vi "hwOperation_GetMeasurementValue.vi"(7 "hwType":string, 8 "Error in":errorcluster, 11 "hwDriverRef in":T1) -> (0 "Error out":errorcluster, 1 "Waveform[]":waveform(dbl)[](array[waveform]), 2 "Time Stamp":timestamp, 3 "hwDriverRef out":T1, 4 "Cluster":cluster{i32[], i32[]}, 5 "Values":dbl[](array[numeric]))   [LabVIEW 2016]
uses:
  QX/hw_QX_hwDriverRef.ctl
  C:/Users/CL/Desktop/ZcDAQprj0811/ZcDAQprj/Modules/DAQ-Device/Hardware Drivers/QX/HBM LabVIEW Driver/DLLs/Hbm.Api.Common.dll
  QX/HBM LabVIEW Driver/DLLs/Hbm.Api.Common.dll
panel:
  in  "Index":i32
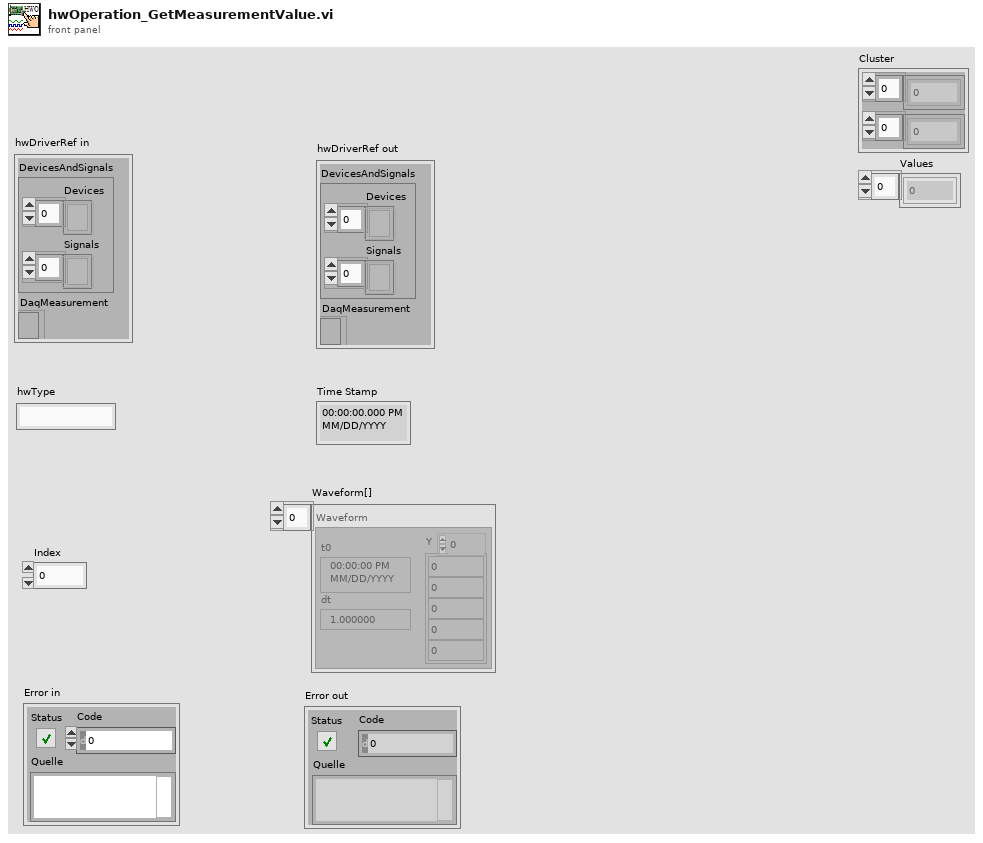
[diagram p1: front panel]
types:
  T1 = typedef "hw_QX_hwDriverRef.ctl" = cluster{"DevicesAndSignals":cluster{"Devices":refnum<k24>[], "Signals":refnum<k24>[]}, "DaqMeasurement":refnum<k24>}
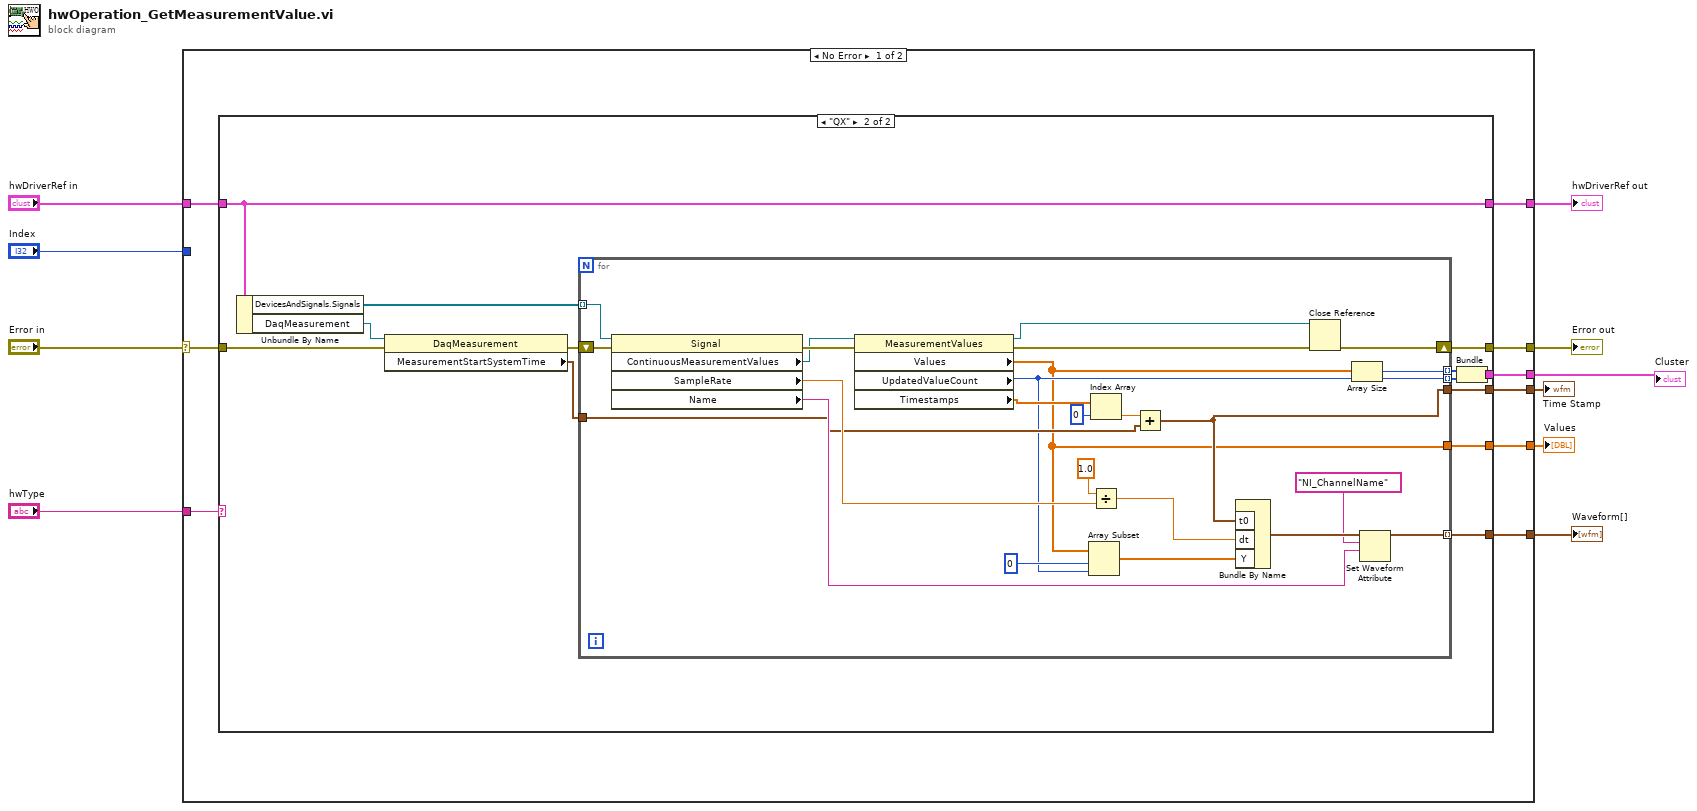
[diagram p0: block diagram]
diagram:
  n1 = case shown="No Error" "Error in" {
    selector: "Error in" -> [w18 w60]
    tunnel: "hwDriverRef in" -> [w19 w59]
    tunnel: [w16 w60] -> w9
    tunnel: [w14 w59] -> w8
    tunnel: "Index" -> [_ _]
    tunnel: [w17 _] -> w6
    tunnel: "hwType" -> [w15 _]
    tunnel: [w13 _] -> w3
    tunnel: [w12 _] -> w2
    tunnel: [w11 _] -> w1
    frame No Error {
      n2 = case shown="\"QX\"" w15 {
        tunnel: w19 -> [w20 w28]
        tunnel: w18 -> [w21 w34]
        tunnel: [_ w32] -> w17
        tunnel: [w21 w31] -> w16
        tunnel: [w20 w28] -> w14
        tunnel: [_ w27] -> w13
        tunnel: [_ w24] -> w12
        tunnel: [_ w23] -> w11
        frame "Simulation", Default {
        }
        frame "QX" {
          n3 = Unbundle By Name(w28) -> ("DevicesAndSignals.Signals"=w30:refnum<k24>[], "DaqMeasurement"=w29:refnum<k24>)
          n4 = property on="Eigenschaftsknoten" class="DaqMeasurement"(reference=w29, error in=w34) -> (error out=w33:errorcluster, "MeasurementStartSystemTime"=w22:timestamp)  [unwired: 1 out]
          n5 = for {
            tunnel: [w48] -> w32 mode=indexing
            shift-right: [w44] -> w31
            shift-left: w33 -> [w50]
            tunnel: w30 -> [w42] mode=indexing
            tunnel: w22 -> [w40]
            tunnel: [w38] -> w27
            tunnel: [w36] -> w26 mode=indexing
            tunnel: [w37] -> w25 mode=indexing
            tunnel: [w35] -> w23
            n6 = property on="Eigenschaftsknoten" class="Signal"(reference=w42, error in=w50) -> (error out=w58:errorcluster, "ContinuousMeasurementValues"=w45:refnum<k24>, "SampleRate"=w55:dbl, "Name"=w47:string)  [unwired: 1 out]
            n7 = property on="Eigenschaftsknoten" class="MeasurementValues"(reference=w45, error in=w58) -> (reference out=w43:refnum<k24>, error out=w46:errorcluster, "Values"=w35:dbl[], "UpdatedValueCount"=w37:i32, "Timestamps"=w57:dbl[])
            n8 = Array Subset "Array Subset"(array=w35, index=0 ("Index"), length=w37) -> (w51:dbl[])
            n9 = Index Array(array=w57, index=0 ("Index")) -> (element=w39:dbl)
            n10 = Divide(x=1.0, y=w55) -> (x/y=w53:dbl)
            n11 = Add(x=w39, y=w40) -> (x+y=w38:timestamp)
            n12 = Bundle By Name("t0"=w38, "dt"=w53, "Y"=w51) -> (w49:waveform(dbl))  [unwired: 1 in]
            n13 = Close Reference(reference=w43, error in (no error)=w46) -> (error out=w44:errorcluster)
            n14 = Array Size(array=w35) -> (size(s)=w36:i32)
            n15 = Set Waveform Attribute(5:w47, 6:"NI_ChannelName" ("Channel Name"), 7:w49) -> (3:w48:waveform(dbl))  [unwired: 1 in, 2 out]
          }
          n16 = Bundle(w26, w25) -> (w24:cluster{i32[], i32[]})  [unwired: 1 in]
        }
      }
    }
    frame Error {
    }
  }
  "Error out" <- w9
  "hwDriverRef out" <- w8
  "Waveform[]" <- w6
  "Time Stamp" <- w3
  "Cluster" <- w2
  "Values" <- w1
